vi "MuxSwitchSingle.vi"(7 "MUX address":u32=1 min=1 max=12 step=1, 8 "error in (no error)":errorcluster, 9 "Channel":i32=1 min=1 max=12 step=1, 10 "C1 / C2":i32=1 min=1 max=12 step=1, 11 "GPIBSwitching in":refnum<class "GPIBSwitching.lvclass">) -> (0 "error out":errorcluster, 2 "command string":string, 3 "GPIBSwitching out":refnum<class "GPIBSwitching.lvclass">)   [LabVIEW 2018, in "GPIBSwitching.lvclass"]
uses:
  GPIBSwitching.lvclass
  C:/ProbeTestSoftware2019/itk-strip-sensor-qc/InstrControl/InstrControl.lvclass
  MUX_CommandsGlobal.vi
  InstrControl.lvclass
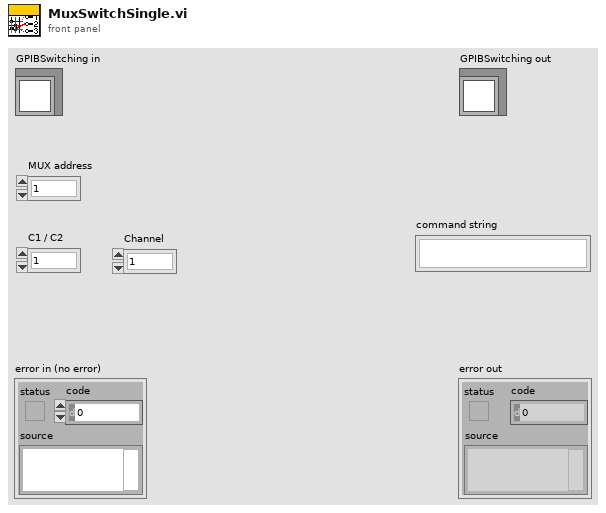
[diagram p1: front panel]
types:
  T1 = cluster{"Mux1 address":string, "Mux2 address":string, "Instrument name":string, "Instrument type":u16, "Command \"MUX Reset\"":string, "Command \"Select MUX Channel\"":string}
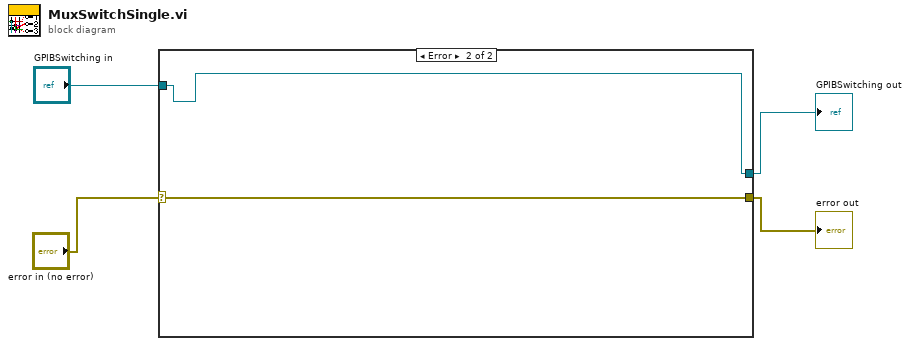
[diagram p0: block diagram]
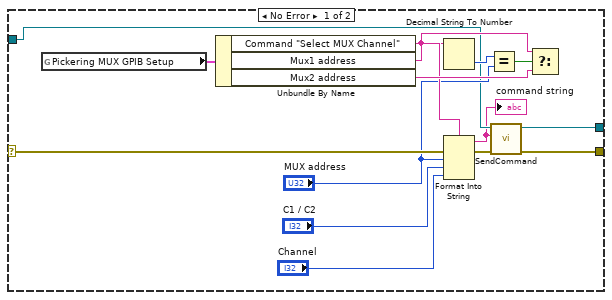
[diagram p2: hidden frame]
diagram:
  n1 = case shown="Error" "error in (no error)" {
    selector: "error in (no error)" -> [w12 w21]
    tunnel: [w11 w21] -> w2
    tunnel: [w10 w20] -> w1
    tunnel: "GPIBSwitching in" -> [w6 w20]
    frame No Error {
      n2 = global read "MUX_CommandsGlobal.vi" "Pickering MUX GPIB Setup"() -> (w19:T1)
      n3 = Unbundle By Name(w19) -> ("Command \"Select MUX Channel\""=w17:string, "Mux1 address"=w14:string, "Mux2 address"=w18:string)
      n4 = Decimal String To Number(string=w14) -> (number=w15:i32)  [unwired: 2 in, 1 out]
      n5 = Format Into String(format string=w17, error in=w12, "MUX address", "C1 / C2", "Channel") -> (resulting string=w5:string, error out=w16:errorcluster)  [unwired: 1 in]
      "command string" <- w5
      n6 = Equal?(x=w15, y="MUX address") -> (x = y?=w13:bool)
      n7 = call "SendCommand.vi"("error in (no error)"=w16, "Command string"=w5, "InstControl in"=w6) -> ("error out"=w11:errorcluster, "InstControl out"=w10:refnum<class "GPIBSwitching.lvclass">)  [unwired: 7 in]
      n8 = Select(t=w14, s=w13, f=w18) -> ()  [unwired: 1 out]
    }
    frame Error {
    }
  }
  "error out" <- w2
  "GPIBSwitching out" <- w1
